vi "Labspec CloseCom.vi"(8 "error in":errorcluster, 11 "Automation Refnum In":refnum<k7>) -> (0 "error out":errorcluster)   [LabVIEW 2014]
panel:
  # "LICENSED MATERIALS – PROPERTY OF IBM\nCopyright IBM Corp. 2016,\nALL RIGHTS RESERVED"
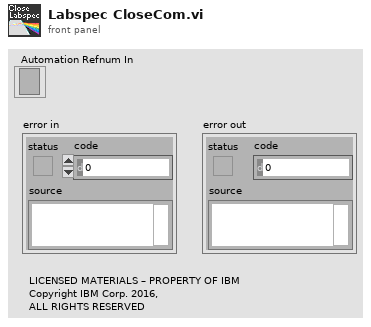
[diagram p1: front panel]
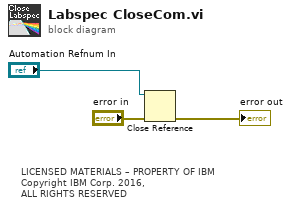
[diagram p0: block diagram]
diagram:
  # "LICENSED MATERIALS – PROPERTY OF IBM\nCopyright IBM Corp. 2016,\nALL RIGHTS RESERVED"
  n1 = Close Reference(reference="Automation Refnum In", error in (no error)="error in") -> (error out=→"error out":errorcluster)
